vi "CNT Get Counter.vi"(7 "pCounterValue":u32, 9 "Channel":u8, 10 "DevIndex":i32, 11 "DevType":i32) -> (3 "function return":i32, 5 "pCounterValue out":u32)   [LabVIEW 2010, in "ControlCNT.lvlib"]
doc: "int WINAPI CNT_GetCounter(int DevType, int DevIndex, unsigned char Channel, unsigned int *pCounterValue);"
uses:
  ControlCNT.lvlib
  ControlCNT/Ginkgo_Driver.dll
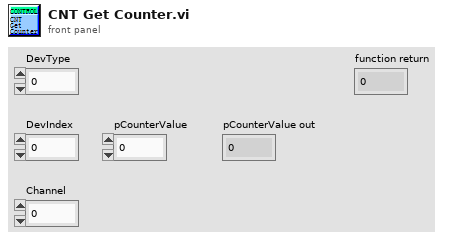
[diagram p1: front panel]
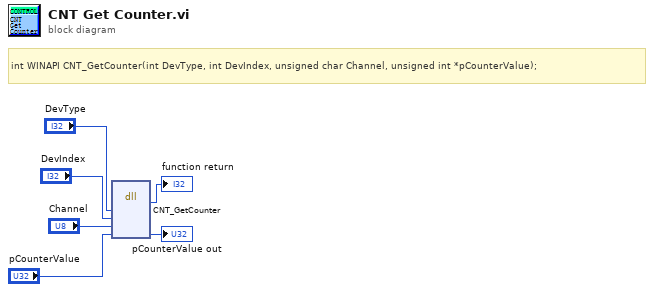
[diagram p0: block diagram]
diagram:
  # "int WINAPI CNT_GetCounter(int DevType, int DevIndex, unsigned char Channel, unsigned int *pCounterValue);"
  n1 = dll-call lib="E:/Project/vt_ginkgo/truck/Ginkgo Driver/vs2010/Ginkgo_USB-I2C&SPI&CAN_API_v2.0.3.3/lib/labview_32bit/ControlCNT/Ginkgo_Driver.*" fn="CNT_GetCounter"("DevType"="DevType", "DevIndex"="DevIndex", "Channel"="Channel", "pCounterValue"="pCounterValue") -> (→"function return":i32, "pCounterValue"=→"pCounterValue out":u32)  [unwired: 6 in, 2 out]
